vi "BitfileSpecific FpgaInterface Creation UserInterface.vi"(11 "Bitfile Path":path) -> ()   [LabVIEW 2010]
doc: "Use this template to build a user interface event handler design pattern. Use this pattern for dialog boxes and other user interfaces. You also can create and execute user-defined events that the VI can handle the same way as user interface events."
uses:
  TypeDefs/FpgaItemToSelect.ctl
  <userlib>/_FPGA Interface Advanced Tools/FPGA Bitfile Utility/TypeDefs/FIFO Info.ctl
  <vilib>/rvi/DataTransferAndStorage/Container/Common/niFpgaDataTypeControl.ctl
  <userlib>/_FPGA Interface Advanced Tools/FPGA Bitfile Utility/TypeDefs/Control_Indicator Info.ctl
  <userlib>/_FPGA Interface Advanced Tools/FPGA Bitfile Utility/FPGA Bitfile Utility.lvlib
panel:
  in  "Deselect All":bool
  in  "Select All":bool
  in  "Cancel":bool
  in  "FPGA Interface Name":string
  in  "Destination Directory":path
  in  "FPGA Items To Add":T1[](array[typedef]) caption="Select FPGA Items to Include in FPGA Interface"
  in  "Generate":bool
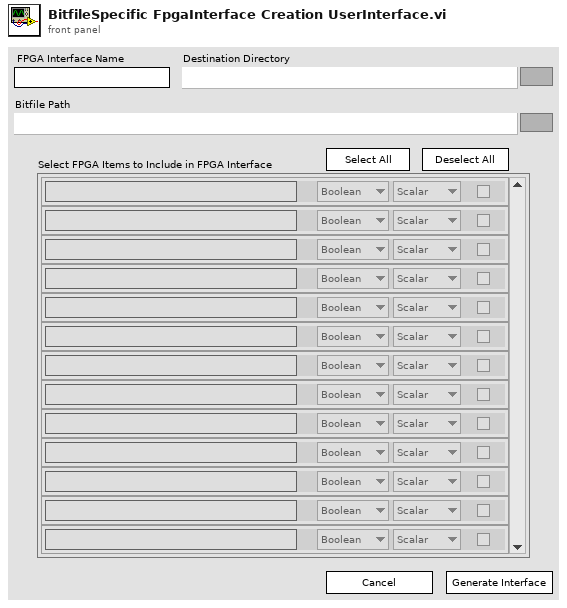
[diagram p1: front panel]
types:
  T1 = typedef "FpgaItemToSelect.ctl" = cluster{"Name":string, "Data Type":enum32{"Boolean", "I8", "I16", "I32", "I64", "U8", "U16", "U32", "U64", "FXP", "CustomControl"}, "Array/Scalar":enum16{"Scalar", "Array", "FIFO"}, "Selected?":bool}
  T2 = typedef "FPGA Bitfile Utility.lvlib/Control_Indicator Info.ctl" = cluster{"Array?":bool, "Data Type":T3, "Address":u32, "Num Elements":u32, "Name":string}
  T3 = typedef "niFpgaDataTypeControl.ctl" = enum32{"Boolean", "I8", "I16", "I32", "I64", "U8", "U16", "U32", "U64", "FXP", "CustomControl"}
  T4 = typedef "FPGA Bitfile Utility.lvlib/FIFO Info.ctl" = cluster{"Data Type":T3, "Physical Channel":u32, "Name":string}
  T5 = enum8{"Enabled", "Disabled", "Disabled and Grayed Out"}
  T6 = cluster{"Control Ref":refnum<vi>, "ClassID":u32, "Name":string, "VI Reference":refnum<vi>}[]
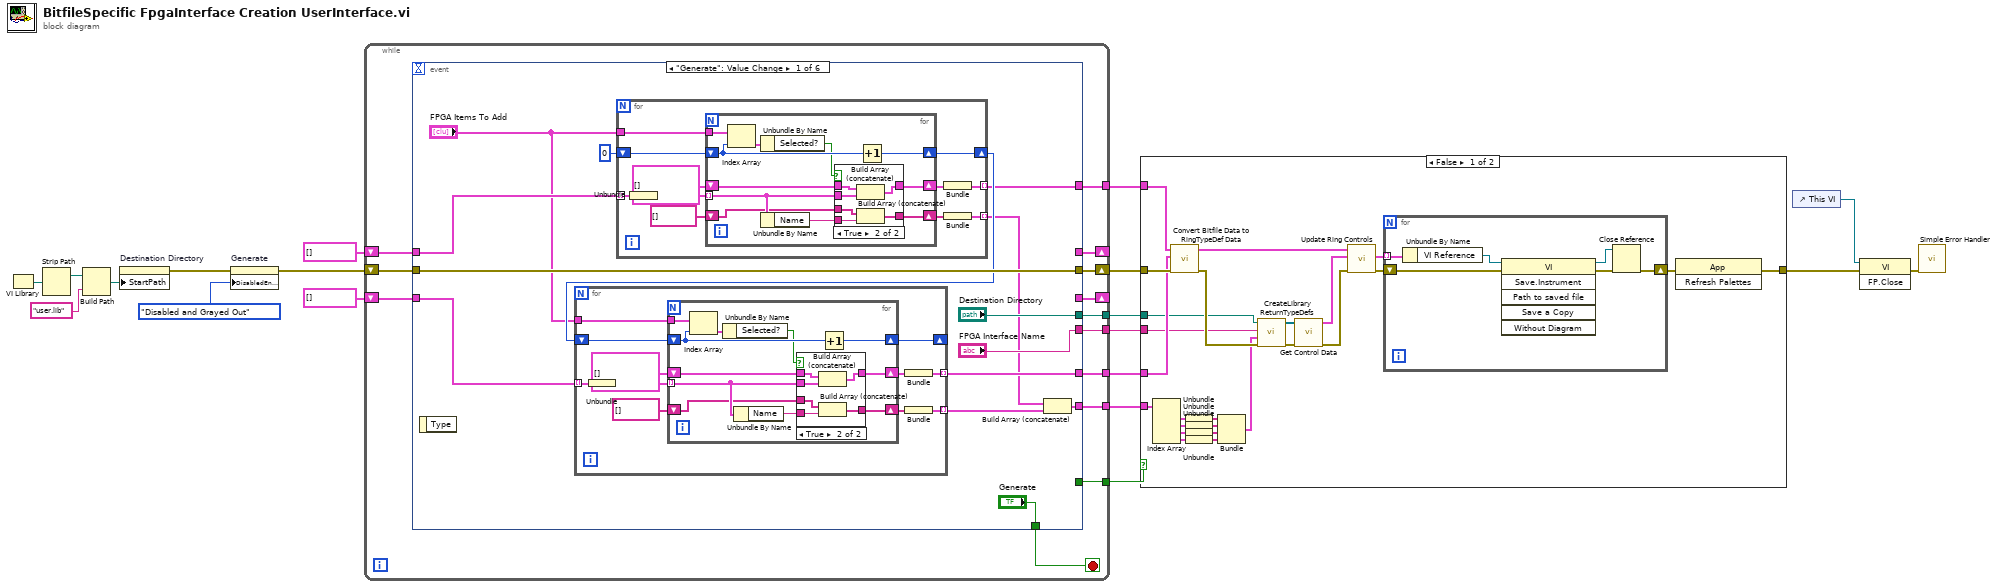
[diagram p0: block diagram]
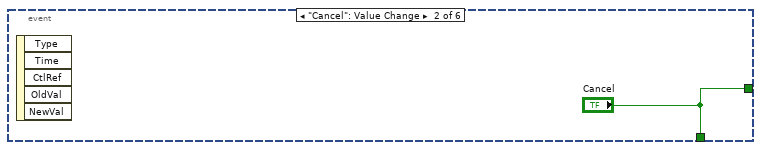
[diagram p5: hidden frame]
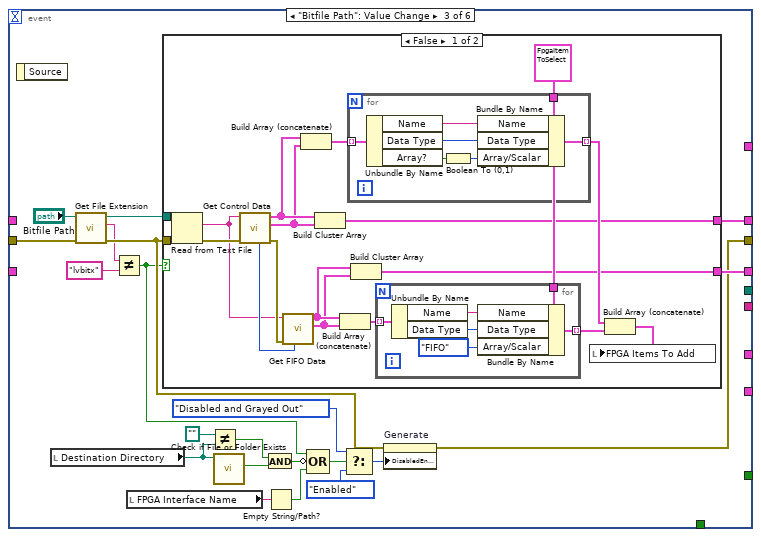
[diagram p6: hidden frame]
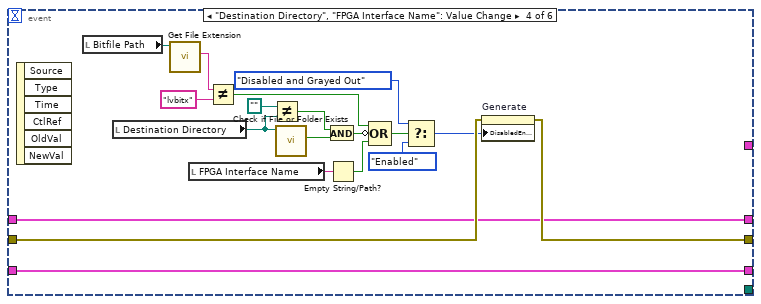
[diagram p8: hidden frame]
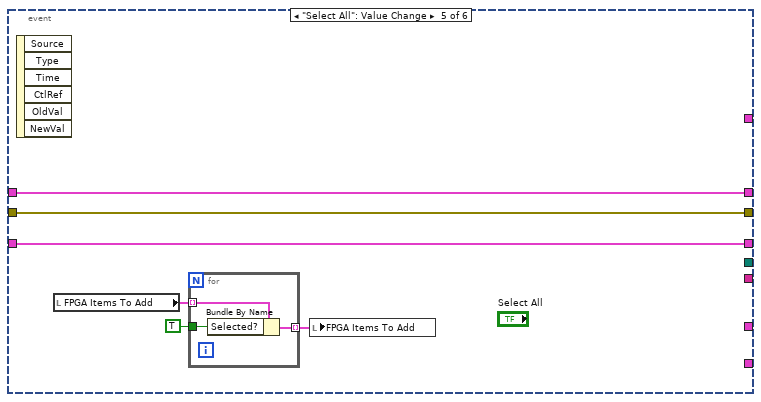
[diagram p9: hidden frame]
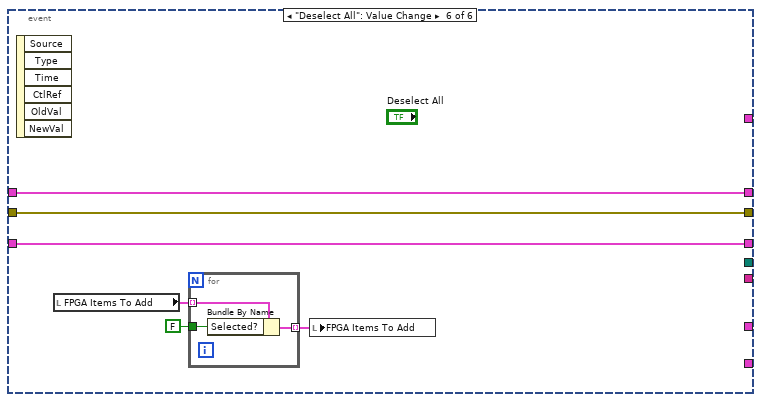
[diagram p10: hidden frame]
diagram:
  n1 = VI Library() -> (path=w5:path)
  n2 = Strip Path(path=w5) -> (stripped path=w4:path)  [unwired: 1 out]
  n3 = Build Path(base path=w4, name or relative path="user.lib") -> (appended path=w2:path)
  n4 = property on="Destination Directory" class="Path"("StartPath"=w2) -> (error out=w1:errorcluster)  [unwired: 2 in, 1 out]
  n5 = property on="Generate" class="Bool"(error in=w1, "DisabledEnum"=T5."Disabled and Grayed Out" ("Disabled")) -> (error out=w15:errorcluster)  [unwired: 1 in, 1 out]
  n6 = while {
    shift-right: [w30] -> w19
    shift-left: w15 -> [w31]
    shift-right: [w26] -> _
    shift-left: cluster{"Controls":T2[]}[] [] -> [w28]
    shift-right: [w29] -> _
    shift-left: cluster{"HostToTargetFIFOs":T4[]}[] [] -> [w27]
    tunnel: [w25] -> w16
    tunnel: [w24] -> w18
    tunnel: [w23] -> w17
    tunnel: [w22] -> w11
    tunnel: [w21] -> w10
    tunnel: [w20] -> w9
    stop <- w32 stop-if-true
    n7 = event shown="[0] \"Generate\": Value Change" {
      selector: _ -> [_ _ _ _ _ _]
      dyn-events: _ -> [_ _ _ _ _ _]
      timeout: _ -> [_ _ _ _ _ _]
      tunnel: ["Generate" "Cancel" _ _ _ _] -> w32
      tunnel: w31 -> [w45 _ w118 w178 w179 w188]
      tunnel: [w45 _ w120 w177 w179 w188] -> w30
      tunnel: [_ _ w127 w176 w183 w192] -> w29
      tunnel: w28 -> [w44 _ _ w175 w184 w193]
      tunnel: w27 -> [w40 _ _ w176 w183 w192]
      tunnel: [_ _ w128 w175 w184 w193] -> w26
      tunnel: [_ "Cancel" _ _ _ _] -> w25
      tunnel: ["Destination Directory" _ _ _ _ _] -> w24
      tunnel: ["FPGA Interface Name" _ _ _ _ _] -> w23
      tunnel: [w37 _ _ _ _ _] -> w22
      tunnel: [w36 _ _ _ _ _] -> w21
      tunnel: [w33 _ _ _ _ _] -> w20
      event "Generate": Value Change {
        n8 = event-data() -> ()  [unwired: 1 in, 1 out]
        n9 = for {
          tunnel: w44 -> [w87] mode=indexing
          shift-right: [w84] -> w42
          shift-left: 0 -> [w86]
          tunnel: "FPGA Items To Add" -> [w85]
          tunnel: [w79] -> w37 mode=indexing
          tunnel: [w77] -> w35 mode=indexing
          n10 = Unbundle(w87) -> ("Controls"=w82:T2[])
          n11 = for {
            tunnel: w82 -> [w91] mode=indexing
            shift-right: [w98] -> w84
            shift-left: w86 -> [w97]
            tunnel: w85 -> [w96]
            shift-right: [w94] -> w81
            shift-left: T2[] [] -> [w93]
            shift-right: [w89] -> w78
            shift-left: string[] [] -> [w88]
            n12 = Index Array(array=w96, index=w97) -> (element=w95:T1)
            n13 = Unbundle By Name(w95) -> ("Selected?"=w92:bool)
            n14 = Unbundle By Name(w91) -> ("Name"=w90:string)
            n15 = case shown="True" w92 {
              tunnel: w91 -> [_ w106]
              tunnel: [w100 w104] -> w94
              tunnel: w93 -> [w100 w105]
              tunnel: w90 -> [_ w103]
              tunnel: [w99 w102] -> w89
              tunnel: w88 -> [w99 w101]
              frame False {
              }
              frame True {
                n16 = Build Array (concatenate)(w105, w106) -> (w104:T2[])
                n17 = Build Array (concatenate)(w101, w103) -> (w102:string[])
              }
            }
            n18 = Increment(x=w97) -> (x+1=w98:i32)
          }
          n19 = Bundle(w81) -> (w79:cluster{T2[]})  [unwired: 1 in]
          n20 = Bundle(w78) -> (w77:cluster{string[]})  [unwired: 1 in]
        }
        n21 = for {
          tunnel: w40 -> [w57] mode=indexing
          shift-right: [w54] -> _
          shift-left: w42 -> [w56]
          tunnel: "FPGA Items To Add" -> [w55]
          tunnel: [w51] -> w36 mode=indexing
          tunnel: [w47] -> w34 mode=indexing
          n22 = Unbundle(w57) -> ("HostToTargetFIFOs"=w52:T4[])
          n23 = for {
            tunnel: w52 -> [w61] mode=indexing
            shift-right: [w68] -> w54
            shift-left: w56 -> [w67]
            tunnel: w55 -> [w66]
            shift-right: [w64] -> w50
            shift-left: T4[] [] -> [w63]
            shift-right: [w59] -> w48
            shift-left: string[] [] -> [w58]
            n24 = Index Array(array=w66, index=w67) -> (element=w65:T1)
            n25 = Unbundle By Name(w65) -> ("Selected?"=w62:bool)
            n26 = Unbundle By Name(w61) -> ("Name"=w60:string)
            n27 = case shown="True" w62 {
              tunnel: w61 -> [_ w76]
              tunnel: [w70 w74] -> w64
              tunnel: w63 -> [w70 w75]
              tunnel: w60 -> [_ w73]
              tunnel: [w69 w72] -> w59
              tunnel: w58 -> [w69 w71]
              frame False {
              }
              frame True {
                n28 = Build Array (concatenate)(w75, w76) -> (w74:T4[])
                n29 = Build Array (concatenate)(w71, w73) -> (w72:string[])
              }
            }
            n30 = Increment(x=w67) -> (x+1=w68:i32)
          }
          n31 = Bundle(w50) -> (w51:cluster{T4[]})  [unwired: 1 in]
          n32 = Bundle(w48) -> (w47:cluster{string[]})  [unwired: 1 in]
        }
        n33 = Build Array (concatenate)(w35, w34) -> (w33:cluster{string[]}[])
      }
      event "Cancel": Value Change {
        n34 = event-data() -> ()  [unwired: 1 in, 5 out]
      }
      event "Bitfile Path": Value Change {
        n35 = event-data() -> ()  [unwired: 1 in, 1 out]
        n36 = local read "Destination Directory"() -> (w110:path)
        n37 = call <vilib>:"Get File Extension.vi"("error in (no error)"=w118, "file"="Bitfile Path") -> ("error out"=w117:errorcluster, "lowercase file extension"=w115:string, "dup file"=w116:path)  [unwired: 6 in, 1 out]
        n38 = Not Equal?(x=w115, y="lvbitx") -> (x != y?=w113:bool)
        n39 = local read "FPGA Interface Name"() -> (w126:string)
        n40 = case shown="False" w113 {
          tunnel: [w134 _] -> w128
          tunnel: [w131 _] -> w127
          tunnel: w117 -> [w130 _]
          tunnel: w116 -> [w129 _]
          frame False {
            w140 = T1 {"Name"="", "Data Type"=enum."Boolean", "Array/Scalar"=enum."Scalar", "Selected?"=TRUE} ("FPGA Item To Select")
            n41 = Read from Text File(file (use dialog)=w129, error in=w130) -> (text=w143:string, error out=w146:errorcluster)  [unwired: 4 out]
            n42 = call <userlib>:"Get Control Data.vi"("error in (no error)"=w146, "bitfile xml in"=w143) -> ("error out"=w144:errorcluster, "Controls"=w135:T2[], "Indicators"=w136:T2[], "offset past EndTag"=w145:i32)  [unwired: 6 in]
            n43 = call <userlib>:"Get FIFO Data.vi"("offset"=w145, "error in (no error)"=w144, "bitfile xml in"=w143) -> ("HostToTargetFIFOs"=w132:T4[], "TargetToHost FIFOs"=w133:T4[])  [unwired: 5 in, 2 out]
            n44 = Build Array (concatenate)(w136, w135) -> (w142:T2[])
            n45 = Build Cluster Array(w136, w135) -> (w134:cluster{"Controls":T2[]}[])
            n46 = Build Array (concatenate)(w133, w132) -> (w141:T4[])
            n47 = for {
              tunnel: w142 -> [w159] mode=indexing
              tunnel: w140 -> [w154]
              tunnel: [w153] -> w139 mode=indexing
              n48 = Unbundle By Name(w159) -> ("Name"=w158:string, "Data Type"=w157:T3, "Array?"=w156:bool)
              n49 = Boolean To (0,1)(Boolean=w156) -> (0, 1=w155:i16)
              n50 = Bundle By Name(cluster=w154, "Name"=w158, "Data Type"=w157, "Array/Scalar"=w155) -> (w153:T1)
            }
            n51 = Build Cluster Array(w133, w132) -> (w131:cluster{"HostToTargetFIFOs":T4[]}[])
            n52 = for {
              tunnel: w141 -> [w152] mode=indexing
              tunnel: w140 -> [w150]
              tunnel: [w147] -> w138 mode=indexing
              n53 = Unbundle By Name(w152) -> ("Name"=w151:string, "Data Type"=w149:T3)
              n54 = Bundle By Name(cluster=w150, "Name"=w151, "Data Type"=w149, "Array/Scalar"=enum16{"Scalar", "Array", "FIFO"}."FIFO") -> (w147:T1)
            }
            n55 = Build Array (concatenate)(w139, w138) -> (w137:T1[])
            n56 = local write "FPGA Items To Add"(w137) -> ()
          }
          frame True {
          }
        }
        n57 = Not Equal?(x=path "", y=w110) -> (x != y?=w109:bool)
        n58 = call <vilib>:"Check if File or Folder Exists.vi"("path"=w110) -> ("file or folder exists?"=w111:bool)  [unwired: 8 in, 2 out]
        n59 = And(x=w109, y=w111) -> (x .and. y?=w112:bool)
        n60 = Empty String/Path?(string/path=w126) -> (empty?=w125:bool)
        n61 = Compound Arithmetic op=OR(w113, invert w112, w125) -> (w124:bool)
        n62 = Select(t=T5."Disabled and Grayed Out" ("Disabled"), s=w124, f=T5."Enabled" ("Disabled")) -> (s? t:f=w123:T5)
        n63 = property on="Generate" class="Bool"(error in=w117, "DisabledEnum"=w123) -> (error out=w120:errorcluster)  [unwired: 1 in, 1 out]
      }
      event "Destination Directory", "FPGA Interface Name": Value Change {
        n64 = event-data() -> ()  [unwired: 1 in, 6 out]
        n65 = local read "Bitfile Path"() -> (w174:path)
        n66 = local read "Destination Directory"() -> (w171:path)
        n67 = call <vilib>:"Get File Extension.vi"("file"=w174) -> ("lowercase file extension"=w166:string)  [unwired: 7 in, 3 out]
        n68 = local read "FPGA Interface Name"() -> (w161:string)
        n69 = Not Equal?(x=w166, y="lvbitx") -> (x != y?=w168:bool)
        n70 = Not Equal?(x=path "", y=w171) -> (x != y?=w172:bool)
        n71 = call <vilib>:"Check if File or Folder Exists.vi"("path"=w171) -> ("file or folder exists?"=w170:bool)  [unwired: 8 in, 2 out]
        n72 = And(x=w172, y=w170) -> (x .and. y?=w169:bool)
        n73 = Empty String/Path?(string/path=w161) -> (empty?=w162:bool)
        n74 = Compound Arithmetic op=OR(w168, invert w169, w162) -> (w163:bool)
        n75 = Select(t=T5."Disabled and Grayed Out" ("Disabled"), s=w163, f=T5."Enabled" ("Disabled")) -> (s? t:f=w160:T5)
        n76 = property on="Generate" class="Bool"(error in=w178, "DisabledEnum"=w160) -> (error out=w177:errorcluster)  [unwired: 1 in, 1 out]
      }
      event "Select All": Value Change {
        n77 = event-data() -> ()  [unwired: 1 in, 6 out]
        n78 = local read "FPGA Items To Add"() -> (w182:T1[])
        n79 = for {
          tunnel: w182 -> [w187] mode=indexing
          tunnel: TRUE ("Selected?") -> [w186]
          tunnel: [w185] -> w180 mode=indexing
          n80 = Bundle By Name(cluster=w187, "Selected?"=w186) -> (w185:T1)
        }
        n81 = local write "FPGA Items To Add"(w180) -> ()
      }
      event "Deselect All": Value Change {
        n82 = event-data() -> ()  [unwired: 1 in, 6 out]
        n83 = local read "FPGA Items To Add"() -> (w191:T1[])
        n84 = for {
          tunnel: w191 -> [w196] mode=indexing
          tunnel: FALSE ("Selected?") -> [w195]
          tunnel: [w194] -> w189 mode=indexing
          n85 = Bundle By Name(cluster=w196, "Selected?"=w195) -> (w194:T1)
        }
        n86 = local write "FPGA Items To Add"(w189) -> ()
      }
    }
  }
  n87 = case shown="False" w16 {
    tunnel: w19 -> [w221 w228]
    tunnel: w18 -> [w197 _]
    tunnel: w17 -> [w199 _]
    tunnel: w11 -> [w212 _]
    tunnel: w10 -> [w211 _]
    tunnel: w9 -> [w210 _]
    tunnel: [w198 w228] -> w6
    frame False {
      n88 = Index Array(array=w210) -> (element #1=w206:cluster{string[]}, element #2=w207:cluster{string[]}, element #3=w208:cluster{string[]}, element #4=w209:cluster{string[]})  [unwired: 4 in]
      n89 = call "Convert Bitfile Data to RingTypeDef Data.vi"("error in"=w221, "FIFOs"=w211, "Registers"=w212) -> ("error out"=w213:errorcluster, "TypeDef Info"=w214:cluster{string, string[]}[])  [unwired: 7 in]
      n90 = Unbundle(w206) -> (w205:string[])
      n91 = Unbundle(w207) -> (w204:string[])
      n92 = Unbundle(w208) -> (w203:string[])
      n93 = Unbundle(w209) -> (w202:string[])
      n94 = Bundle(w205, w204, w203, w202) -> (w201:cluster{string[], string[], string[], string[]})  [unwired: 1 in]
      n95 = call "CreateLibrary ReturnTypeDefs.vi"("error in (no error)"=w213, "Names of Registers"=w201, "New Name"=w199, "Destination Directory"=w197) -> ("error out"=w217:errorcluster, "TypeDef Refs"=w218:refnum<vi>[])  [unwired: 5 in, 1 out]
      n96 = call <userlib>:"Get Control Data.vi"("error in (no error)"=w217, "TypeDef Refs"=w218) -> ("error out"=w220:errorcluster, "Control Data"=w219:T6)  [unwired: 8 in]
      n97 = call "Update Ring Controls.vi"("error in (no error)"=w220, "Control Data"=w219, "Parsed Header Data"=w214) -> ("error out"=w215:errorcluster, "Control Data Out"=w216:T6)  [unwired: 7 in]
      n98 = for {
        tunnel: w216 -> [w227] mode=indexing
        shift-right: [w223] -> w200
        shift-left: w215 -> [w226]
        n99 = Unbundle By Name(w227) -> ("VI Reference"=w222:refnum<vi>)
        n100 = invoke class="VI" method="Save.Instrument"(reference=w222, error in=w226) -> (reference out=w224:refnum<vi>, error out=w225:errorcluster)  [unwired: 4 in, 4 out]
        n101 = Close Reference(reference=w224, error in (no error)=w225) -> (error out=w223:errorcluster)
      }
      n102 = invoke class="App" method="Refresh Palettes"(error in=w200) -> (error out=w198:errorcluster)  [unwired: 2 in, 2 out]
    }
    frame True {
    }
  }
  n103 = control-ref of="This VI"() -> (w7:refnum<vi>)
  n104 = invoke class="VI" method="FP.Close"(reference=w7, error in=w6) -> (error out=w8:errorcluster)  [unwired: 1 in, 2 out]
  n105 = call <vilib>:"Simple Error Handler.vi"("error in (no error)"=w8) -> ()  [unwired: 4 in, 5 out]
